vi "send PVUpdate.vi"(8 "error in (no error)":errorcluster, 9 "PV":refnum<class "PV.lvclass">, 10 "CS++PVUpdate Msg in":refnum<class "CS++PVUpdate Msg.lvclass">, 11 "Message Enqueuer in":refnum<class "Message Enqueuer.lvclass">) -> (0 "error out":errorcluster, 3 "Message Enqueuer out":refnum<class "Message Enqueuer.lvclass">)   [LabVIEW 2013, in "CS++PVMonitor.lvlib" / "CS++PVUpdate Msg.lvclass"]
uses:
  CS++PVUpdate Msg.lvclass
  Classes/CS++ProcessVariables/ProcessVariable/PV.lvclass
  <vilib>/ActorFramework/Message Enqueuer/Message Enqueuer.lvclass
  CS++PVUpdate Msg.lvclass/CS++PVUpdate Msg.ctl
  <vilib>/ActorFramework/Message Enqueuer/Message Enqueuer.lvclass/Message Enqueuer.ctl
  <vilib>/ActorFramework/Message Priority Queue/Priority Enqueue.vi
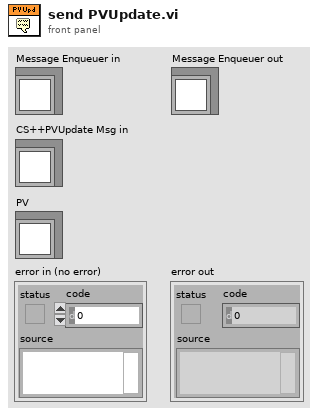
[diagram p1: front panel]
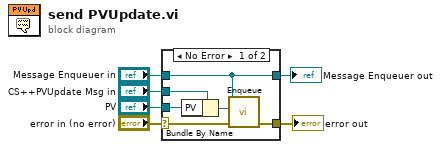
[diagram p0: block diagram]
diagram:
  n1 = case shown="No Error" "error in (no error)" {
    selector: "error in (no error)" -> [w9 w14]
    tunnel: [w8 w14] -> w5
    tunnel: "CS++PVUpdate Msg in" -> [w11 _]
    tunnel: "PV" -> [w12 _]
    tunnel: "Message Enqueuer in" -> [w7 w13]
    tunnel: [w7 w13] -> w1
    frame No Error {
      n2 = Bundle By Name(cluster=w11, "PV"=w12) -> (w10:refnum<class "CS++PVUpdate Msg.lvclass">)
      n3 = call <vilib>:"Enqueue.vi"("error in (no error)"=w9, "Message"=w10, "Message Enqueuer in"=w7) -> ("error out"=w8:errorcluster)  [unwired: 7 in, 1 out]
    }
    frame Error {
    }
  }
  "error out" <- w5
  "Message Enqueuer out" <- w1
